vi "Write BG color.vi"(8 "error in (no error)":errorcluster, 10 "BG color":i32, 11 "Picture in":refnum<class "Picture.lvclass">) -> (0 "error out":errorcluster, 3 "Picture out":refnum<class "Picture.lvclass">)   [LabVIEW 2018, in "Picture.lvclass"]
uses:
  Picture.lvclass
  Picture.lvclass/Picture.ctl
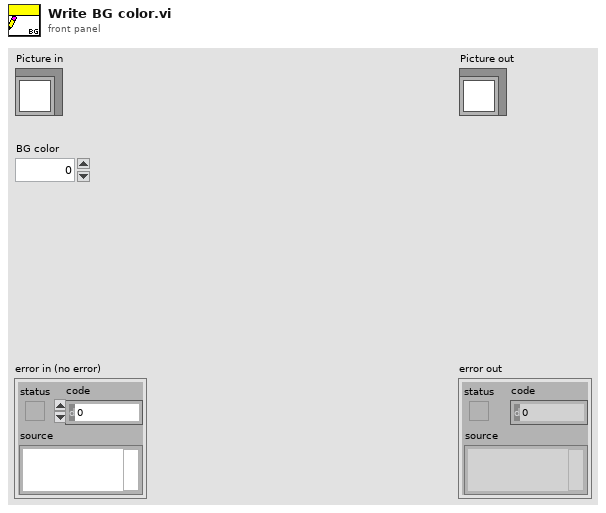
[diagram p1: front panel]
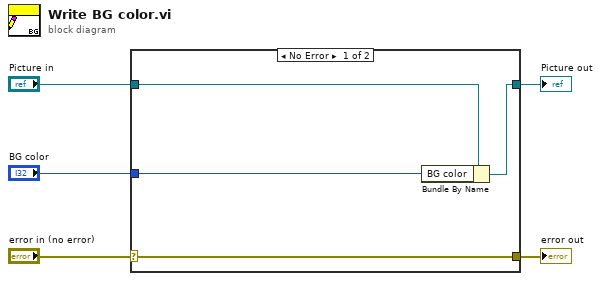
[diagram p0: block diagram]
diagram:
  n1 = case shown="No Error" "error in (no error)" {
    selector: "error in (no error)" -> [w9 w10]
    tunnel: [w9 w10] -> w4
    tunnel: [w7 w11] -> w2
    tunnel: "Picture in" -> [w8 w11]
    tunnel: "BG color" -> [w6 _]
    frame No Error {
      n2 = Bundle By Name(cluster=w8, "BG color"=w6) -> (w7:refnum<class "Picture.lvclass">)
    }
    frame Error {
    }
  }
  "error out" <- w4
  "Picture out" <- w2
